vi "server.vi"() -> ()   [LabVIEW 2019]
uses:
  <vilib>/NI/STM/SubVIs/MetaDataElement.ctl
  <vilib>/NI/STM/TCP/Write Meta Data (TCP Ref).vi
  b6e12540-0c00-4818-8e74-44bb0aade04b.vi
  <vilib>/NI/STM/TCP/Get Connection Reference (TCP).vi
  <vilib>/NI/STM/TCP/Write Meta Data (TCP Clst).vi
  <vilib>/NI/STM/TCP/Read Message (TCP).vi
  <vilib>/NI/STM/TCP/Write Message (TCP).vi
  <vilib>/NI/STM/NI STM.lvlib
panel:
  in  "name":enum16{"Start", "CMD"}(ring)
  in  "MOVE Command":T1
  out "error  out":errorcluster
  in  "stop":bool
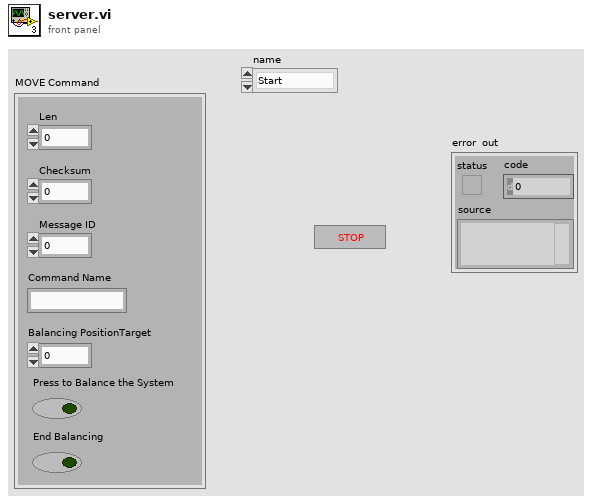
[diagram p1: front panel]
types:
  T1 = cluster{"Len":u8, "Checksum":u16, "Message ID":u16, "Command Name":string, "Balancing PositionTarget ":dbl, "Press to Balance the System":bool, "End Balancing":bool}
  T2 = typedef "NI STM.lvlib/MetaDataElement.ctl" = string
  T3 = typedef "NI STM.lvlib/TCP Connection Info.ctl" = cluster{"connection ID":refnum<k5>, "meta data":T2[]}
  T4 = cluster{"Len":u8, "Checksum":u16, "Message ID":u16, "Command Name":u32, "Balancing PositionTarget ":dbl, "Press to Balance the System":bool, "End Balancing":bool}
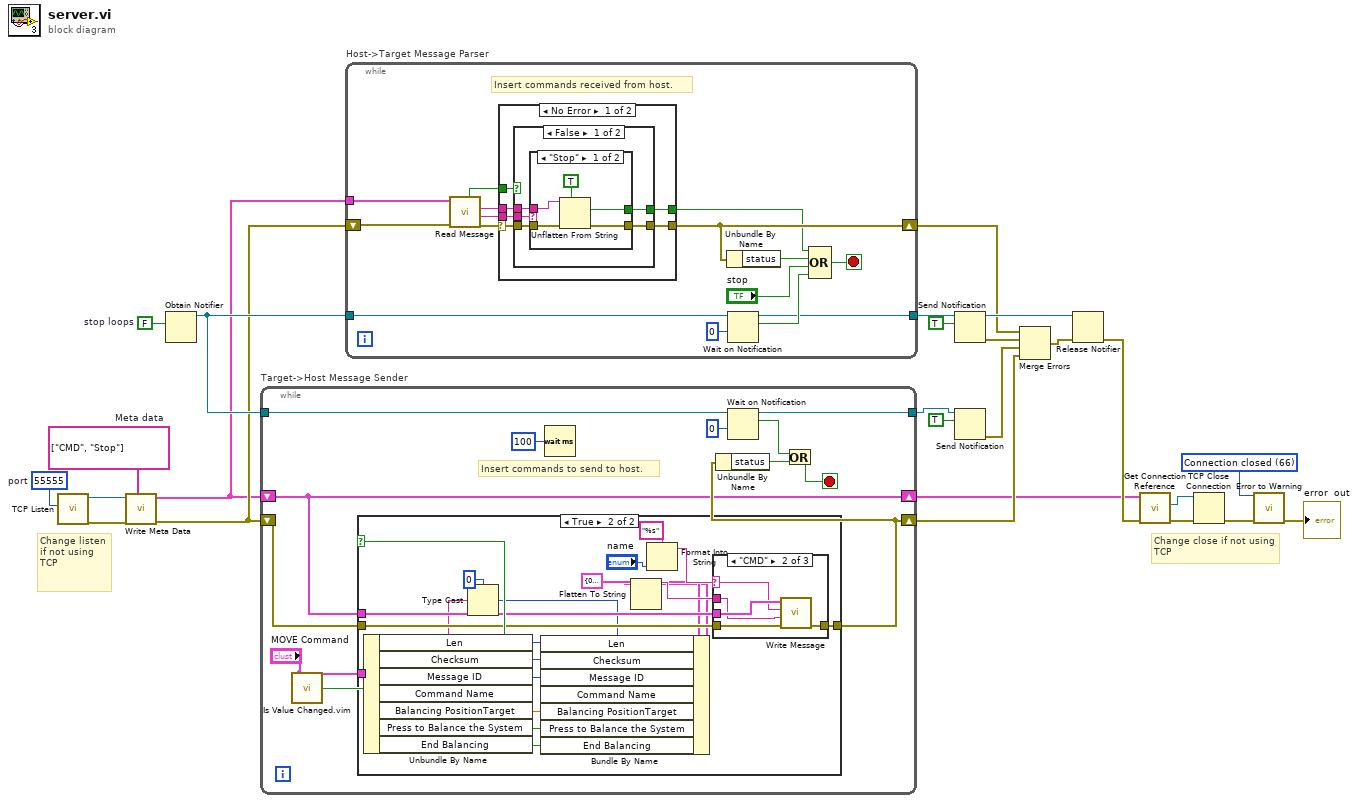
[diagram p0: block diagram]
diagram:
  w11 = FALSE  # stop loops
  w1 = T2[] ["CMD", "Stop"]  # Meta data
  w23 = 66 items=["No Error", "Argument Error", "Memory Full", "Out of Zone", "End of File", "File Already Open", "Generic File IO Error", "File Not Found", "File Permission Error", "Disk Full", "Duplicate Path", "Too Many Files Open", "Not Enabled", "Resource File Not Found", "Cannot Add Resource", "Resource Not Found", "Image Not Found", "Image Memory Error", "Pen Does Not Exist", "Config Bad Type", "Config Token Not Found", "Config Parse Error", "Config Memory Error", "Bad External Code Format", "Bad External Code Offset", "External Code Not Present", "Null Window", "Destroy Window Mixup", "Null Menu", "Print Aborted", "Bad Print Record", "Print Driver Error", "Windows Error During Print", "Memory Error During Print", "Print Dialog Error", "Generic Print Error", "Invalid Device Refnum", "Device Not Found", "Device Parameter Error", "Device Unit Error", "Can't Open Device", "Device Call Aborted", "Generic Error", "Cancelled By User", "Object ID Too Low", "Object ID Too High", "Object Not In Heap", "Unknown Heap", "Bad DefProc ID", "DefProc Not In Table", "Message Out Of Range", "Null Method", "Unknown Message", "Manager Call Not Supported", "Bad address", "Connection In progress", "Connection timed out", "Connection is already in progress", "Network attribute not supported", "Network error", "Address in use", "System out of memory", "Connection aborted", "Connection refused", "Connection is not connected", "Connection is already connected", "Connection closed", "Initialize error (interapplication manager)", "Bad occurrence", "Wait on unbound occurrence handler", "Occurrence queue overflow", "Bad path", "Semaphore not signaled", "Unrecognized type (interapplication manager)"] ("1st Error to Convert")
  w2 = u16 55555  # port
  # "Change close if not using TCP"
  # "Change listen if not using TCP"
  n1 = call <vilib>:"TCP Listen.vi"("port"=w2) -> ("error out"=w3:errorcluster, "connection ID"=w10:refnum<k5>)  [unwired: 3 in, 6 out]
  n2 = call-poly <vilib>:"Write Meta Data.vi"("meta data"=w1, "error in"=w3, "connection ID"=w10) -> ("error out"=w5:errorcluster, "connection info out"=w4:T3)  [unwired: 2 in, 5 out]
  n3 = Obtain Notifier(notification data type=w11) -> (notifier out=w14:refnum<notifier>)  [unwired: 3 in, 2 out]
  n4 = while "Target->Host Message Sender" {
    shift-right: [w28] -> w19
    shift-left: w5 -> [w29]
    shift-right: [w27] -> w6
    shift-left: w4 -> [w27]
    tunnel: w14 -> [w36]
    tunnel: [w32] -> w16
    stop <- w33 stop-if-true
    # "Insert commands to send to host."
    n5 = call "Is Value Changed.vim"("value"="MOVE Command") -> ("changed or first call?"=w30:bool)
    n6 = case shown="True" w30 {
      tunnel: w27 -> [_ w57]
      tunnel: w29 -> [w38 w56]
      tunnel: [w38 w55] -> w28
      tunnel: "MOVE Command" -> [_ w45]
      frame False {
      }
      frame True {
        n7 = Unbundle By Name(w45) -> ("Len"=w44:u8, "Checksum"=w43:u16, "Message ID"=w42:u16, "Command Name"=w49:string, "Balancing PositionTarget"=w41:dbl, "Press to Balance the System"=w40:bool, "End Balancing"=w39:bool)
        n8 = Type Cast(type=u32 0, x=w49) -> (*(type *) &x=w50:u32)
        n9 = Bundle By Name(cluster=T4 {"Len"=0, "Checksum"=0, "Message ID"=0, "Command Name"=0, "Balancing PositionTarget "=0.0, "Press to Balance the System"=FALSE, "End Balancing"=FALSE} ("MOVE Command 2"), "Len"=w44, "Checksum"=w43, "Message ID"=w42, "Command Name"=w50, "Balancing PositionTarget"=w41, "Press to Balance the System"=w40, "End Balancing"=w39) -> (w46:T4)
        n10 = Flatten To String(anything=w46) -> (data string=w54:string)  [unwired: 3 in, 2 out]
        n11 = Format Into String(format string="%s", "name") -> (resulting string=w52:string)  [unwired: 2 in, 1 out]
        n12 = case shown="\"CMD\"" w52 {
          selector: w52 -> [_ w60 _]
          tunnel: w57 -> [_ w63 _]
          tunnel: w56 -> [w58 w62 w64]
          tunnel: [w58 w61 w64] -> w55
          tunnel: w54 -> [_ w59 _]
          frame Default {
          }
          frame "CMD" {
            n13 = call-poly <vilib>:"Write Message.vi"("error in"=w62, "data"=w59, "name"=w60, "connection info in"=w63) -> ("error out"=w61:errorcluster)  [unwired: 6 in, 1 out]
          }
          frame "STA" {
          }
        }
      }
    }
    n14 = Wait (ms)(milliseconds to wait=u32 100) -> ()  [unwired: 1 out]
    n15 = Unbundle By Name(w28) -> ("status"=w34:bool)
    n16 = Wait on Notification(notifier=w36, timeout in ms (-1)=0) -> (notifier out=w32:refnum<notifier>, notification=w35:bool)  [unwired: 2 in, 2 out]
    n17 = Or(x=w35, y=w34) -> (x .or. y?=w33:bool)
  }
  n18 = while "Host->Target Message Parser" {
    tunnel: w4 -> [w79]
    shift-right: [w71] -> w9
    shift-left: w5 -> [w78]
    tunnel: w14 -> [w72]
    tunnel: [w67] -> w13
    stop <- w66 stop-if-true
    # "Insert commands received from host."
    n19 = call-poly <vilib>:"Read Message.vi"("error in"=w78, "connection info in"=w79) -> ("error out"=w74:errorcluster, "name"=w77:T2, "data string"=w76:string, "timed out?"=w75:bool)  [unwired: 3 in, 3 out]
    n20 = case shown="No Error" w74 {
      selector: w74 -> [w82 w98]
      tunnel: w77 -> [w85 _]
      tunnel: w76 -> [w84 _]
      tunnel: w75 -> [w83 _]
      tunnel: [w81 w98] -> w71
      tunnel: [w80 _] -> w65
      frame No Error {
        n21 = case shown="False" w83 {
          tunnel: w85 -> [w87 _]
          tunnel: w84 -> [w90 _]
          tunnel: w82 -> [w89 w97]
          tunnel: [w88 w97] -> w81
          tunnel: [w86 _] -> w80
          frame False {
            n22 = case shown="\"Stop\"" w87 {
              tunnel: w90 -> [w94 _]
              tunnel: w89 -> [w93 w96]
              tunnel: [w91 w96] -> w88
              tunnel: [w92 _] -> w86
              frame "Stop" {
                n23 = Unflatten From String(type=TRUE, binary string=w94, error in (no error)=w93) -> (value=w92:bool, error out=w91:errorcluster)  [unwired: 1 in, 2 out]
              }
              frame Default {
              }
            }
          }
          frame True {
          }
        }
      }
      frame Error {
      }
    }
    n24 = Unbundle By Name(w71) -> ("status"=w70:bool)
    n25 = Wait on Notification(notifier=w72, timeout in ms (-1)=0) -> (notifier out=w67:refnum<notifier>, notification=w68:bool)  [unwired: 2 in, 2 out]
    n26 = Compound Arithmetic op=OR(w65, w70, "stop", w68) -> (w66:bool)
  }
  n27 = Send Notification(notification=TRUE, notifier=w13) -> (notifier out=w20:refnum<notifier>, error out=w17:errorcluster)  [unwired: 1 in]
  n28 = Send Notification(notification=TRUE, notifier=w16) -> (error out=w18:errorcluster)  [unwired: 1 in, 1 out]
  n29 = Merge Errors(w9, w17, w18, w19) -> (w21:errorcluster)
  n30 = Release Notifier(notifier=w20, error in (no error)=w21) -> (error out=w22:errorcluster)  [unwired: 1 in, 2 out]
  n31 = call-poly <vilib>:"Get Connection Reference.vi"("error in"=w22, "connection info in"=w6) -> ("error out"=w8:errorcluster, "connection ID out"=w7:refnum<k5>)  [unwired: 8 out]
  n32 = TCP Close Connection(connection ID=w7, error in (no error)=w8) -> (error out=w24:errorcluster)  [unwired: 2 out]
  n33 = call <vilib>:"Error to Warning.vi"("1st Error to Convert"=w23, "error in"=w24) -> ("warning out"=→"error  out":errorcluster)  [unwired: 3 in, 10 out]
